vi "GetWiresAroundtheselectedNode.vi"(8 "error in (no error)":errorcluster, 10 "Sel Node reference":refnum<vi>, 11 "VI reference In":refnum<vi>) -> (0 "error out":errorcluster, 3 "WiresInRange[]":refnum<vi>[](array[refnum]))   [LabVIEW 2014]
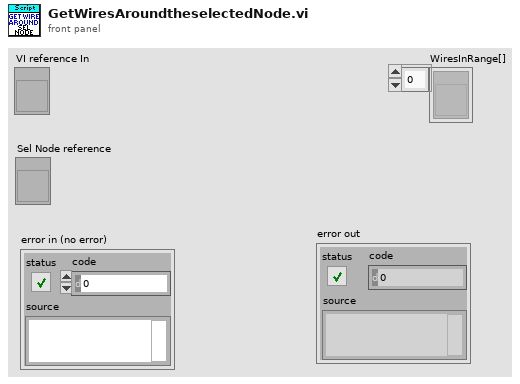
[diagram p1: front panel]
types:
  T1 = typedef "LVRectTypeDef.ctl" = cluster{"Left":i16, "Top":i16, "Right":i16, "Bottom":i16}
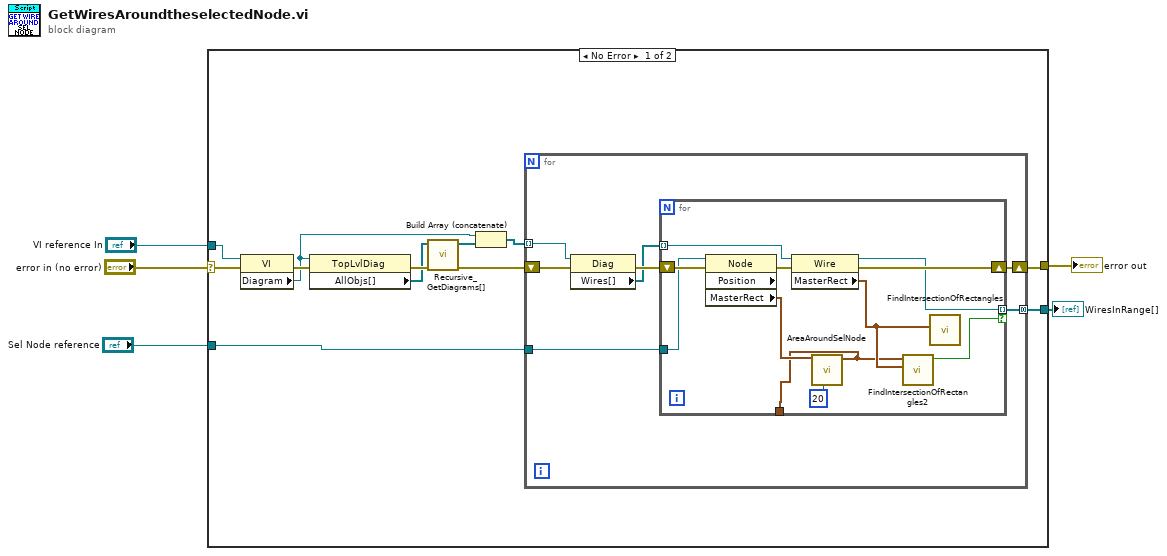
[diagram p0: block diagram]
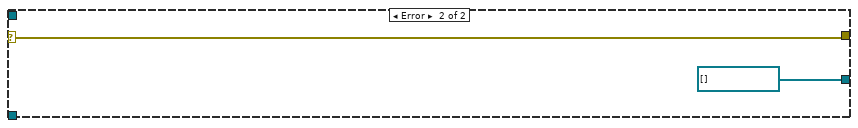
[diagram p2: hidden frame]
diagram:
  n1 = case shown="No Error" "error in (no error)" {
    selector: "error in (no error)" -> [w16 w37]
    tunnel: "VI reference In" -> [w12 _]
    tunnel: [w15 w37] -> w3
    tunnel: "Sel Node reference" -> [w14 _]
    tunnel: [w13 refnum<vi>[] []] -> w1
    frame No Error {
      n2 = property on="Property Node" class="VI"(reference=w12, error in=w16) -> (error out=w17:errorcluster, "Diagram"=w6:refnum<vi>)  [unwired: 1 out]
      n3 = property on="Property Node" class="TopLvlDiag"(reference=w6, error in=w17) -> (error out=w11:errorcluster, "AllObjs[]"=w9:refnum<vi>[])  [unwired: 1 out]
      n4 = call "Recursive_GetDiagrams[].vi"("error in (no error)"=w11, "AllObjs[]"=w9) -> ("error out"=w10:errorcluster, "Diagrams"=w8:refnum<vi>[])  [unwired: 8 in]
      n5 = Build Array (concatenate)(w6, w8) -> (w7:refnum<vi>[])
      n6 = for {
        tunnel: w14 -> [w23]
        tunnel: [w22] -> w13 mode=concatenating
        shift-right: [w24] -> w15
        shift-left: w10 -> [w21]
        tunnel: w7 -> [w19] mode=indexing
        n7 = property class="Diag"(reference=w19, error in=w21) -> (error out=w20:errorcluster, "Wires[]"=w18:refnum<vi>[])  [unwired: 1 out]
        n8 = for {
          tunnel: w18 -> [w31] mode=indexing
          tunnel: w23 -> [w32]
          shift-right: [w33] -> w24
          shift-left: w20 -> [w35]
          tunnel: [w30] -> w22 mode=indexing if=w28
          tunnel: [w25] -> _
          n9 = property on="Property Node" class="Wire"(reference=w31, error in=w35) -> (reference out=w30:refnum<vi>, error out=w34:errorcluster, "MasterRect"=w29:T1)
          n10 = property on="Property Node" class="Node" props=["Position", "MasterRect"](reference=w32, error in=w34) -> (error out=w33:errorcluster, "MasterRect"=w26:T1)  [unwired: 2 out]
          n11 = call "AreaAroundSelNode.vi"("Distance"=i16 20, "Master Bounds Rect"=w26) -> ("Bounds+Distance"=w25:T1)  [unwired: 9 in]
          n12 = call "FindIntersectionOfRectangles2.vi"("Wire"=w29, "Node"=w25) -> ("Intersect?"=w28:bool)  [unwired: 9 in]
          n13 = call "FindIntersectionOfRectangles.vi"("Wire"=w29) -> ()  [unwired: 10 in, 1 out]
        }
      }
    }
    frame Error {
    }
  }
  "error out" <- w3
  "WiresInRange[]" <- w1
